vi "refModelDP3rd.vi"(10 "eta_d":dbl[](array[numeric])) -> (1 "x_r":dbl, 2 "y_r":dbl, 3 "psi_r":dbl)   [LabVIEW 2014]
uses:
  <vilib>/Simulation/Implementation/Shared/SIMSCR Execution Mode.ctl
  <vilib>/Simulation/Scripting/Companion Diagram/SimConfigNode/SimParams.ctl
  <vilib>/Simulation/Scripting/Companion Diagram/SimConfigNode/_simSolvers.ctl
  <vilib>/Simulation/Param Hierarchy/Typedefs/SIMPH Param Control Actions.ctl
  <vilib>/Simulation/Implementation/Shared/SIM limit type.ctl
  <vilib>/Simulation/Implementation/Shared/NILVSim_ParamChanged.vi
  <vilib>/Simulation/Implementation/Shared/NILVSIM_BeginStep.vi
  <vilib>/Simulation/ContinuousLinear/Implementation/NILVSim Integrator new.llb/SIM Integrator Distributor (vector).vi
  <vilib>/Simulation/SignalArithmetic/Implementation/NILVSim Gain.llb/SIM Gain (vector,MatrixGain).vi
  <vilib>/Simulation/Nonlinear/Implementation/NILVSim Saturation.llb/SIM Saturation (vector).vi
  <vilib>/Simulation/ContinuousLinear/Implementation/NILVSim Integrator new.llb/SIM Integrator Collector (vector).vi
  <vilib>/Simulation/Implementation/Shared/NILVSim_Manager.vi
  <vilib>/Utility/error.llb/Clear Errors.vi
  <vilib>/Simulation/Implementation/Shared/NILVSim_FinalizeModel.vi
  <vilib>/Simulation/Implementation/Shared/SIM Unbundle Sim Info.vi
  <vilib>/Simulation/Implementation/Shared/SIMSH Read Queue.vi
  <vilib>/Simulation/Implementation/Shared/NILVSim_Initialize.vi
  <vilib>/Simulation/Utility/Implementation/NILVSim Get Time and IsAcceptedStep.vi
  <vilib>/Simulation/Implementation/Shared/NILVSim_GetModelError.vi
  <vilib>/Simulation/Implementation/Shared/SIM SimErrorHandler.vi
  <vilib>/Simulation/Implementation/Shared/SIM Bundle Sim Info.vi
  <vilib>/Simulation/Scripting/Companion Diagram/SimConfigNode/SimDog.xnode
  <vilib>/Simulation/Implementation/XNodeFramework/SimXNode/SimX.xnode
  <vilib>/Simulation/ContinuousLinear/Implementation/NILVSim Integrator new.llb/SIM Integrator (vector).vi
  <vilib>/Simulation/Implementation/Shared/NI_SIM_Implementation.lvlib
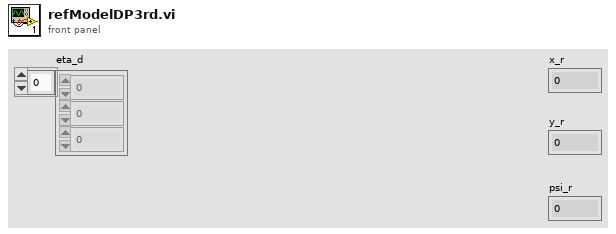
[diagram p1: front panel]
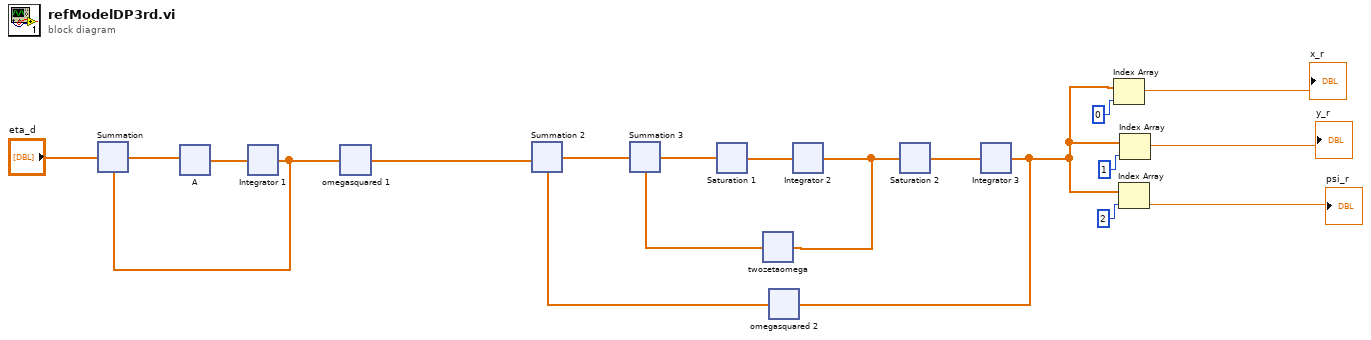
[diagram p0: block diagram]
diagram:
  n1 = xnode "Summation"("Operand1"="eta_d", "Operand2"=w6) -> ("Result"=w19:dbl[])
  n2 = xnode "A"("input"=w19) -> ("output"=w7:dbl[])  [unwired: 3 in]
  n3 = xnode "Integrator 1"("input"=w7) -> ("output"=w6:dbl[])  [unwired: 9 in, 2 out]
  n4 = xnode "omegasquared 1"("input"=w6) -> ("output"=w14:dbl[])  [unwired: 3 in]
  n5 = xnode "Summation 2"("Operand1"=w14, "Operand2"=w16) -> ("Result"=w18:dbl[])
  n6 = xnode "Summation 3"("Operand1"=w18, "Operand2"=w17) -> ("Result"=w15:dbl[])
  n7 = xnode "Saturation 1"("input"=w15) -> ("output"=w5:dbl[])  [unwired: 4 in]
  n8 = xnode "Integrator 2"("input"=w5) -> ("output"=w4:dbl[])  [unwired: 9 in, 2 out]
  n9 = xnode "twozetaomega"("input"=w4) -> ("output"=w17:dbl[])  [unwired: 3 in]
  n10 = xnode "Saturation 2"("input"=w4) -> ("output"=w3:dbl[])  [unwired: 4 in]
  n11 = xnode "Integrator 3"("input"=w3) -> ("output"=w2:dbl[])  [unwired: 9 in, 2 out]
  n12 = xnode "omegasquared 2"("input"=w2) -> ("output"=w16:dbl[])  [unwired: 3 in]
  n13 = Index Array(array=w2, index=0) -> (element=→"x_r":dbl)
  n14 = Index Array ("Index Array 3")(array=w2, index=2 ("index 3")) -> (element=→"psi_r":dbl)
  n15 = Index Array ("Index Array 2")(array=w2, index=1 ("index 2")) -> (element=→"y_r":dbl)
